vi "Lissajous.vi"() -> ()   [LabVIEW 2020]
uses:
  <vilib>/measure/NI_MABase.lvlib
panel:
  out "Waveform Graph":waveform(dbl)(graph)
  out "Voltaje Wave":waveform(dbl)(graph)
  in  "stop":bool
  out "rms Corriente":dbl(knob) scale=0.0..10.0
  out "rms Voltaje":dbl(knob) scale=0.0..10.0
  in  "Corriente":T1 {"Fase" scale=-90.0..90.0; "Frecuencia" scale=0.0..500.0; "Amplitud" scale=0.0..1000.0}
  out "XY Graph":cluster{"Y":dbl[], "Y":dbl[]}(graph)
  in  "Voltaje":T1 {"Fase" scale=-90.0..90.0; "Frecuencia" scale=0.0..500.0; "Amplitud" scale=0.0..1000.0}
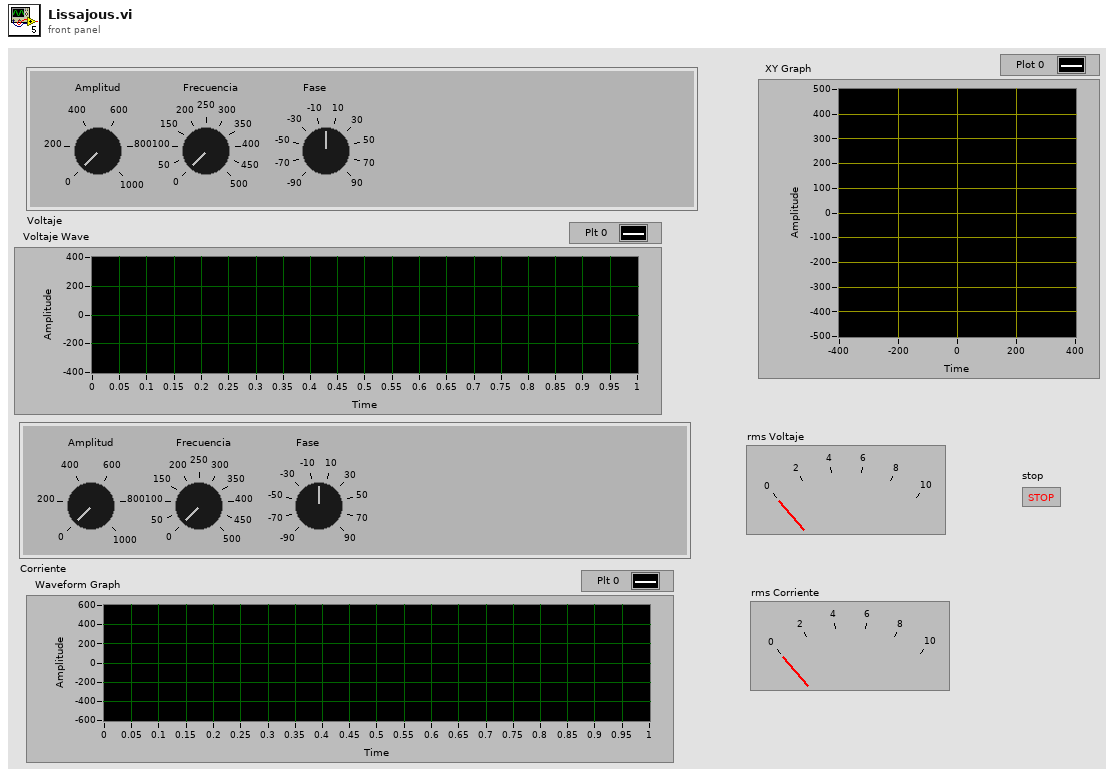
[diagram p1: front panel]
types:
  T1 = cluster{"Amplitud":dbl, "Frecuencia":dbl, "Fase":dbl}
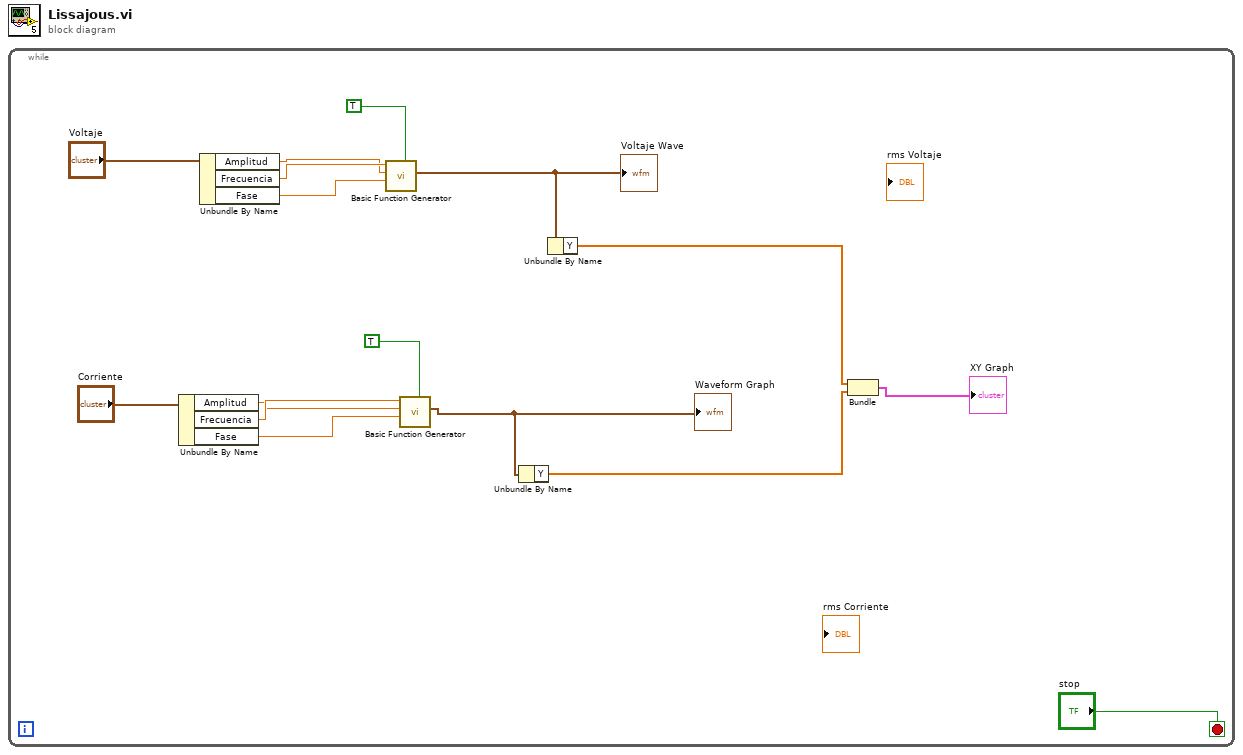
[diagram p0: block diagram]
diagram:
  n1 = while {
    stop <- "stop" stop-if-true
    n2 = Unbundle By Name("Corriente") -> ("Amplitud"=w9:dbl, "Frecuencia"=w10:dbl, "Fase"=w8:dbl)
    n3 = Unbundle By Name("Voltaje") -> ("Amplitud"=w12:dbl, "Frecuencia"=w13:dbl, "Fase"=w11:dbl)
    n4 = call <vilib>:"Basic Function Generator.vi"("reset signal"=TRUE, "phase"=w11, "amplitude"=w12, "frequency"=w13) -> ("signal out"=w5:waveform(dbl))  [unwired: 5 in, 2 out]
    "Voltaje Wave" <- w5
    n5 = call <vilib>:"Basic Function Generator.vi"("reset signal"=TRUE, "phase"=w8, "amplitude"=w9, "frequency"=w10) -> ("signal out"=w2:waveform(dbl))  [unwired: 5 in, 2 out]
    "Waveform Graph" <- w2
    n6 = Unbundle By Name(w2) -> ("Y"=w4:dbl[])
    n7 = Unbundle By Name(w5) -> ("Y"=w1:dbl[])
    n8 = Bundle("Y"=w1, "Y"=w4) -> (→"XY Graph":cluster{"Y":dbl[], "Y":dbl[]})  [unwired: 1 in]
  }
